vi "Main.vi"() -> ()   [LabVIEW 2017]
uses:
  MassData-Parameter/Utility/Def-MassData Status Indicator(Vertical).ctl
  <userlib>/_NEVSTOP/Communicable State Machine(CSM)/_Polymophic/Add State(s) to Queue By BOOL(Element).vi
  92441261-0e8a-4c49-872b-6a8cc16470f8.vi
  cdca145a-d193-4db9-b465-521fbe583cf5.vi
  <vilib>/Analysis/2dsp.llb/Real FFT.vi
  <userlib>/_NEVSTOP/Communicable State Machine(CSM)/AdvanceAPI/CSM - Revert Arguments-Safe String.vi
  <userlib>/_NEVSTOP/Communicable State Machine(CSM)/AdvanceAPI/CSM - Make String Arguments Safe.vi
  <userlib>/_NEVSTOP/Communicable State Machine(CSM)/AdvanceAPI/CSM - Break Down Multiple States String.vi
  <userlib>/_NEVSTOP/Communicable State Machine(CSM)/AdvanceAPI/CSM - Compact Multiple States.vi
  <userlib>/_NEVSTOP/Communicable State Machine(CSM)/AdvanceAPI/CSM - Keywords.vi
  <userlib>/_NEVSTOP/Communicable State Machine(CSM)/_Shared/Trim Single-line Text.vi
  MassData-Parameter/_support/FGV-MassData.vi
  MassData-Parameter/CSM MassData Parameter Support.lvlib
  <vilib>/Analysis/NI_AALPro.lvlib
  <userlib>/_NEVSTOP/Communicable State Machine(CSM)/Communicable State Machine.lvlib
panel:
  out "MassData Status":T1={"w"={287840.0, 276144.0}, "r"={287840.0, 276144.0}} {"r" scale=1.0..1000000.0 scale format="%#_6p"; "w" scale=1.0..1000000.0 scale format="%#_6p"}
  out "fft":dbl[](graph)
  in  "Gen?":bool
  in  "DataSize":i32=1000
  out "Waveform Chart":dbl[](graph)
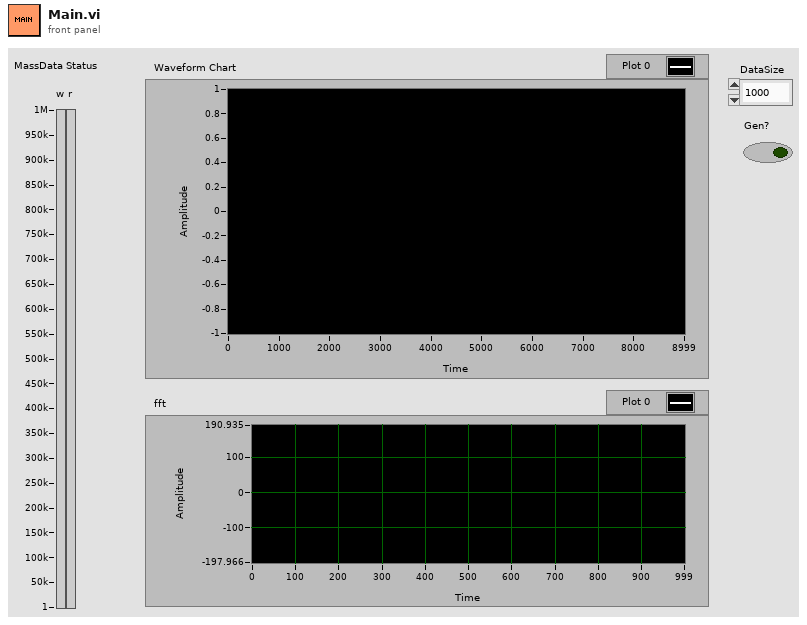
[diagram p1: front panel]
types:
  T1 = typedef "Def-MassData Status Indicator(Vertical).ctl" = cluster{"w":cluster{dbl, dbl}, "r":cluster{dbl, dbl}}
  T2 = enum32{"Invalid", "Standard", "Closed", "Hidden", "Minimized", "Maximized"}
  T3 = enum32{"invalid app kind", "Development System", "Run Time System", "Student Edition", "Embedded LabVIEW", "Evaluation", "Custom"}
  T4 = typedef "Communicable State Machine.lvlib/_CSM_Response Source Message.ctl" = cluster{"‘State":string, "’Arguments":string, "’Error":errorcluster}
  T5 = cluster{"Core":cluster{"Current VI Reference":refnum<vi>, "Close Panel on Exit?":bool}, "Your Boolean data":bool, "Your string data":string}
  T6 = cluster{"Current VI Reference":refnum<vi>, "Close Panel on Exit?":bool}
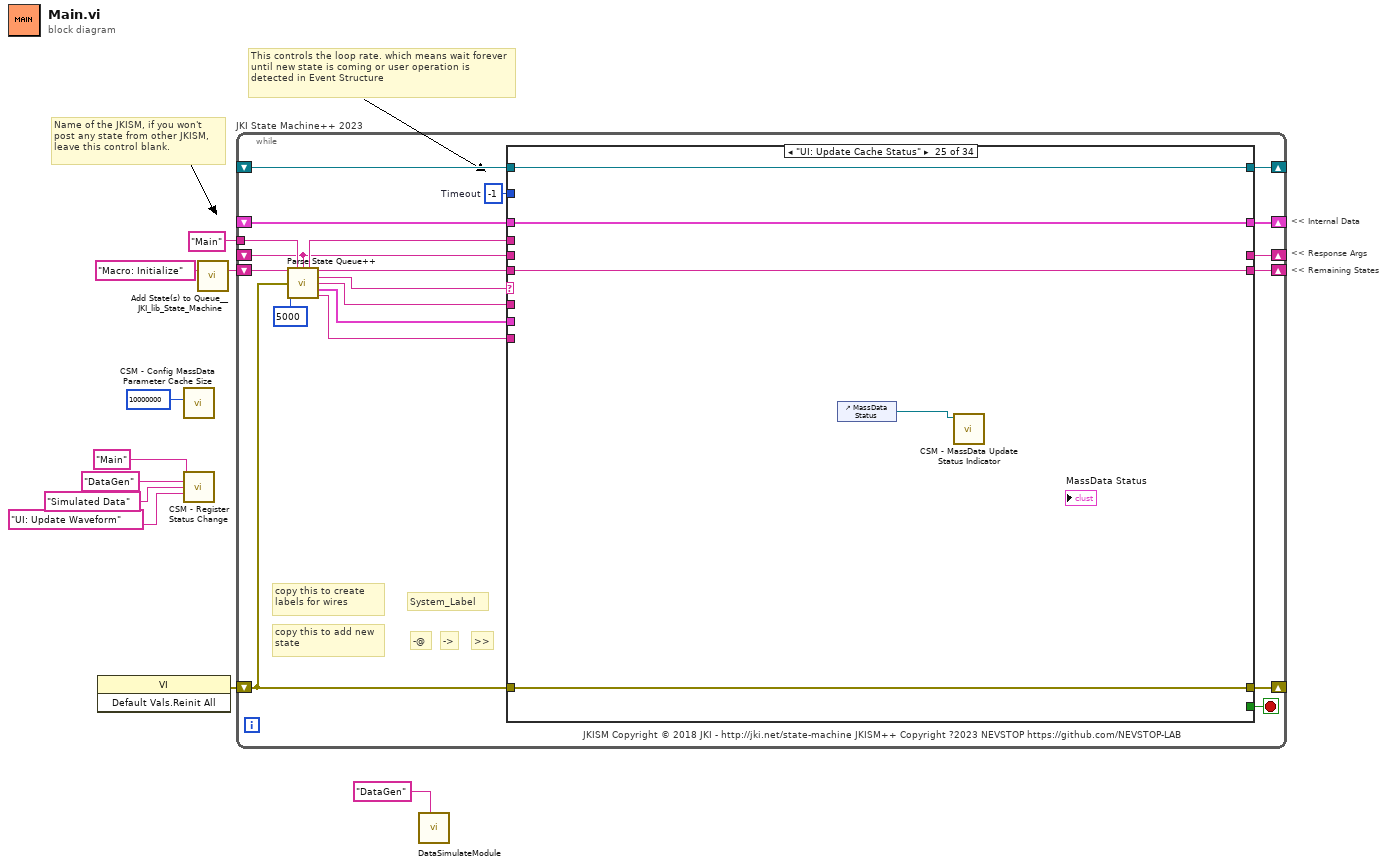
[diagram p0: block diagram]
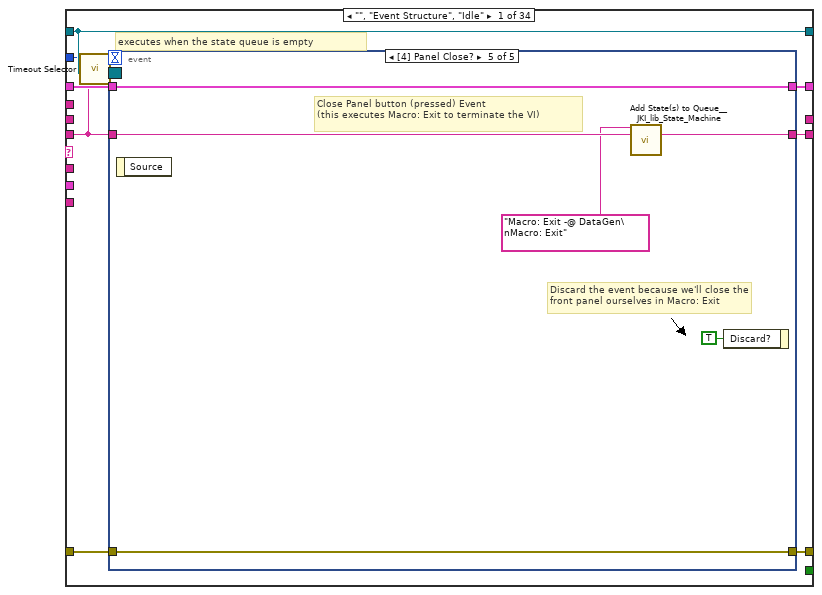
[diagram p2: hidden frame]
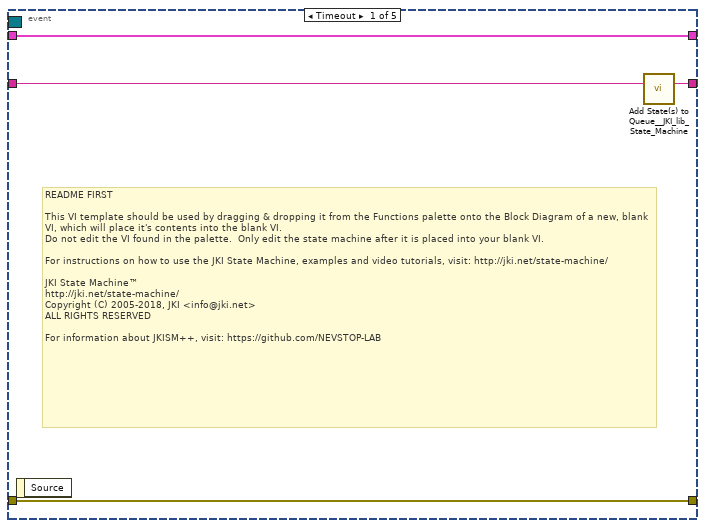
[diagram p3: hidden frame]
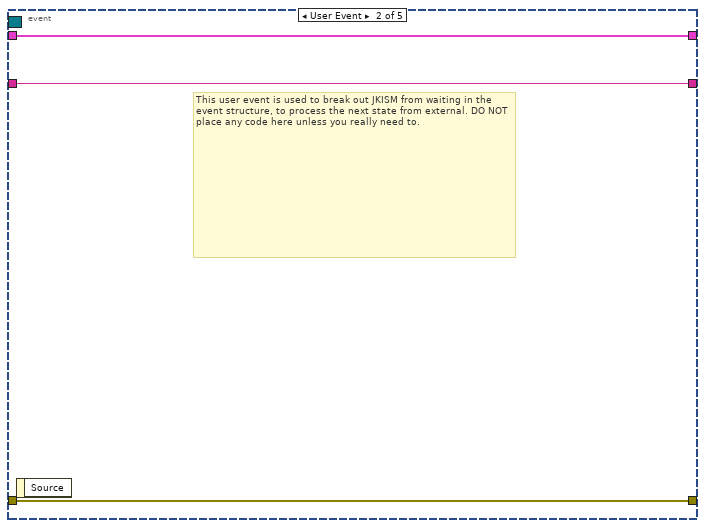
[diagram p4: hidden frame]
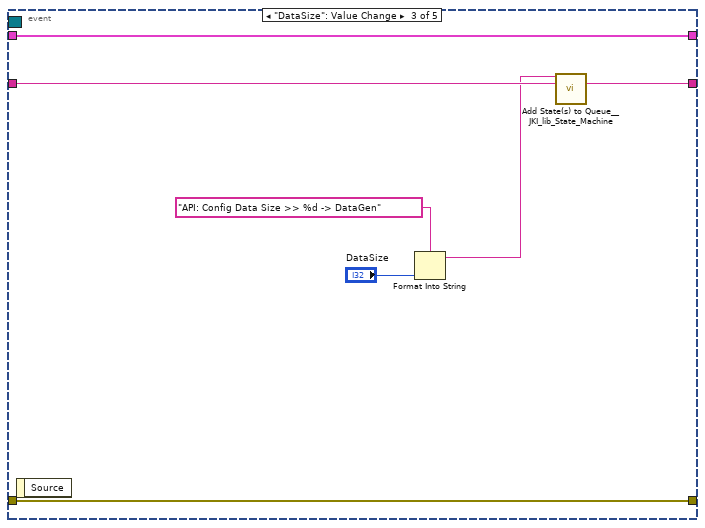
[diagram p5: hidden frame]
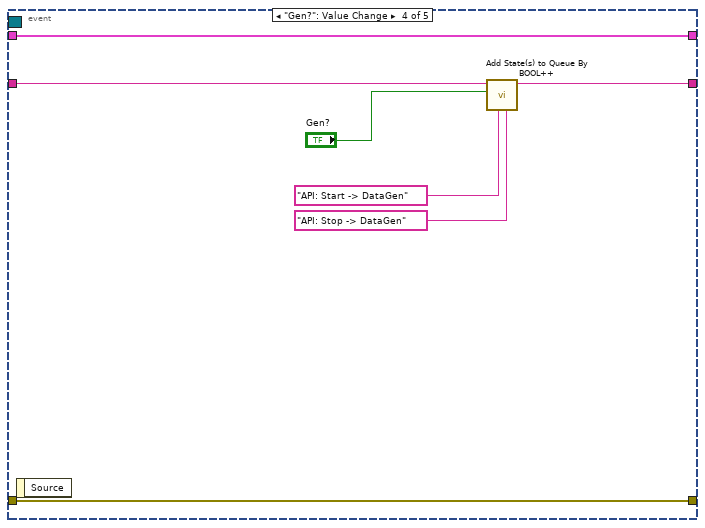
[diagram p6: hidden frame]
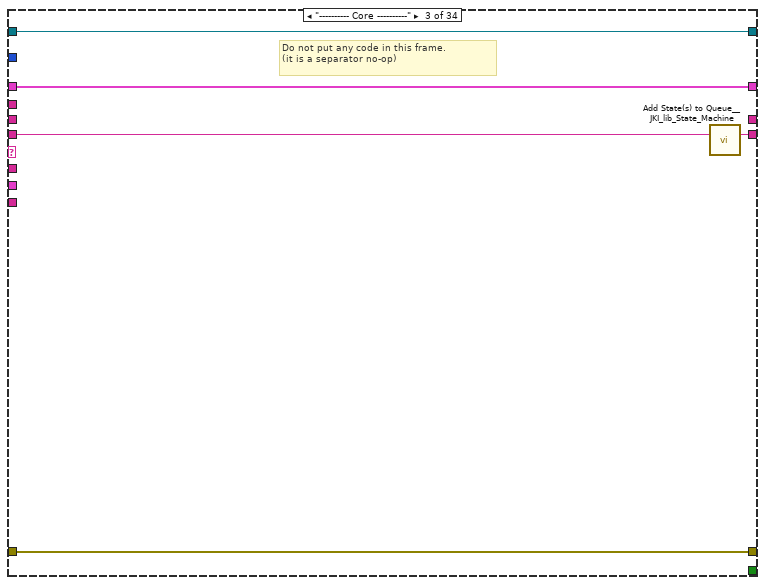
[diagram p8: hidden frame]
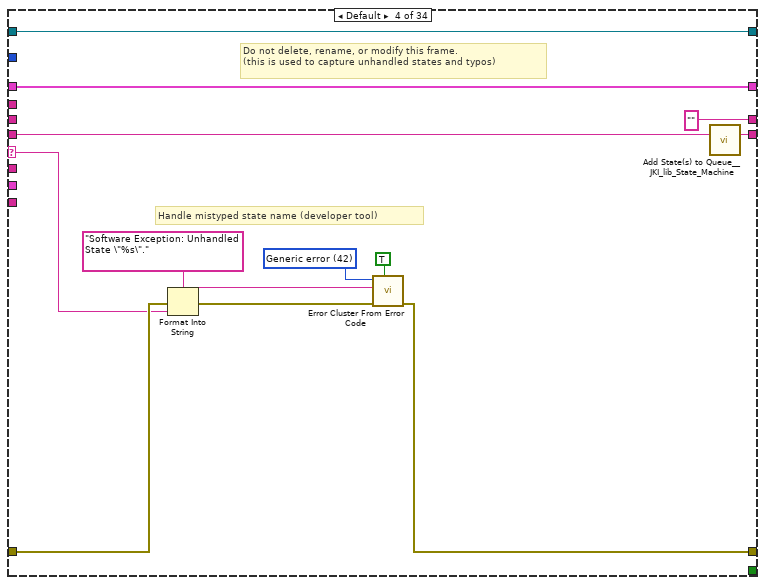
[diagram p9: hidden frame]
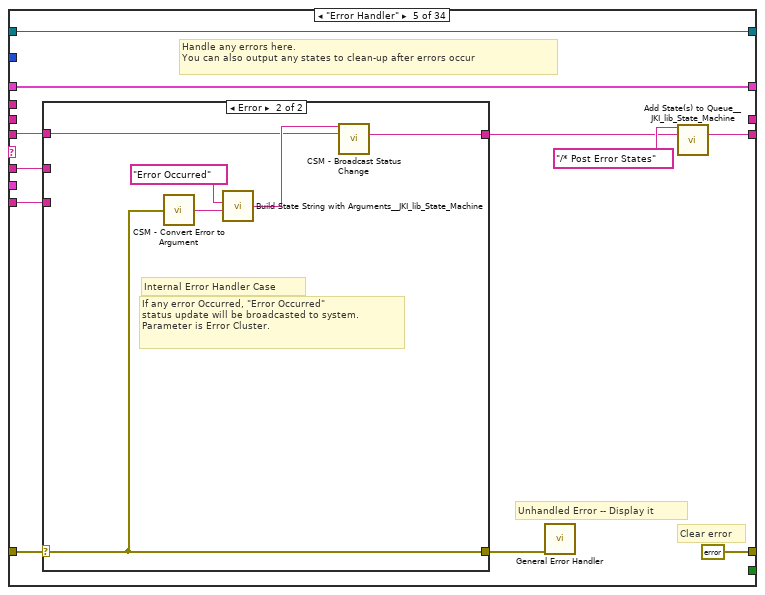
[diagram p10: hidden frame]
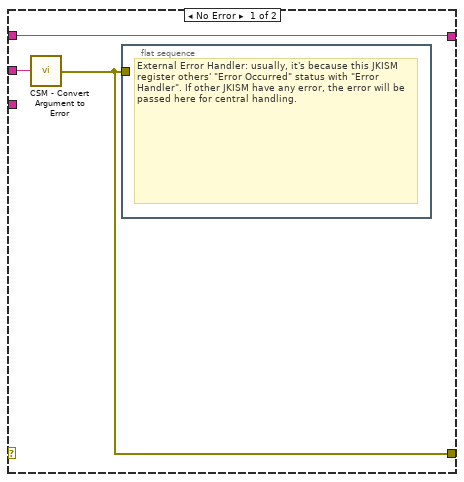
[diagram p11: hidden frame]
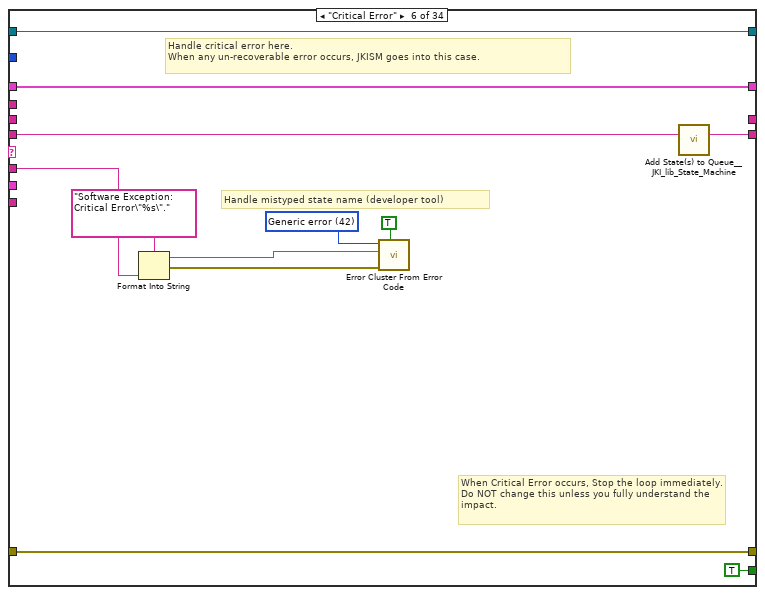
[diagram p12: hidden frame]
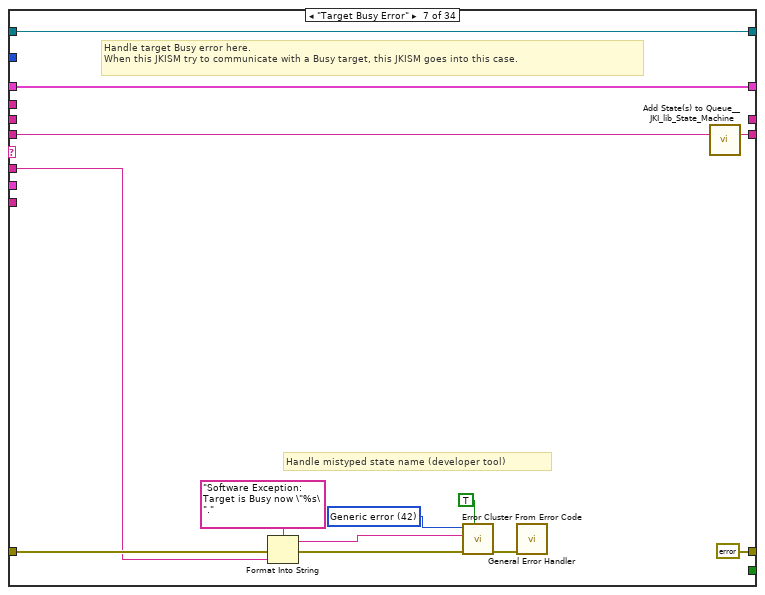
[diagram p13: hidden frame]
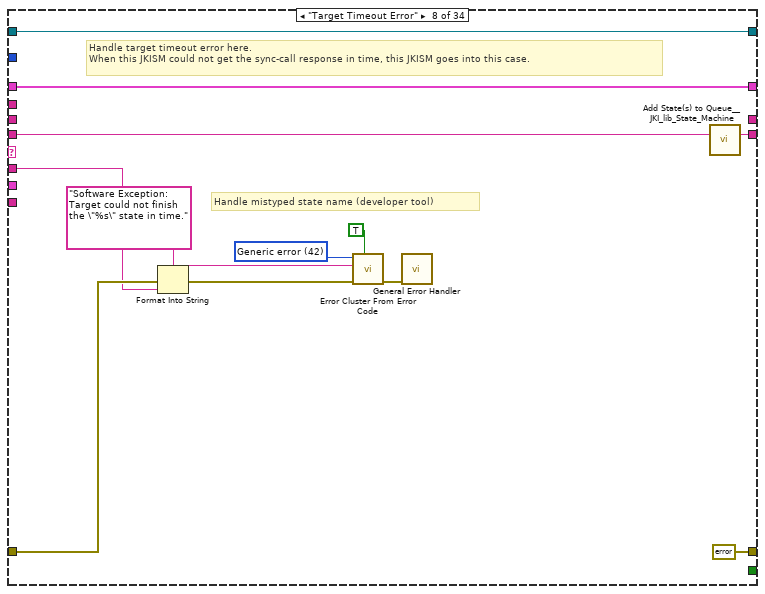
[diagram p14: hidden frame]
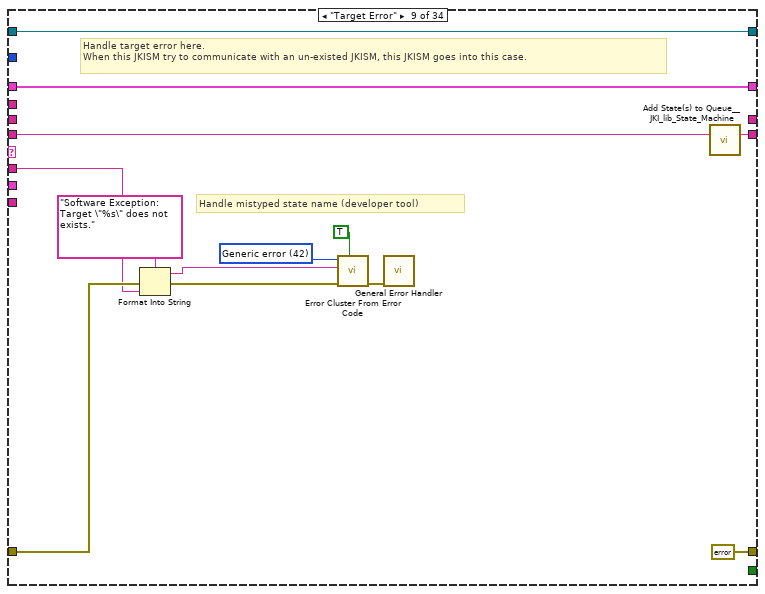
[diagram p15: hidden frame]
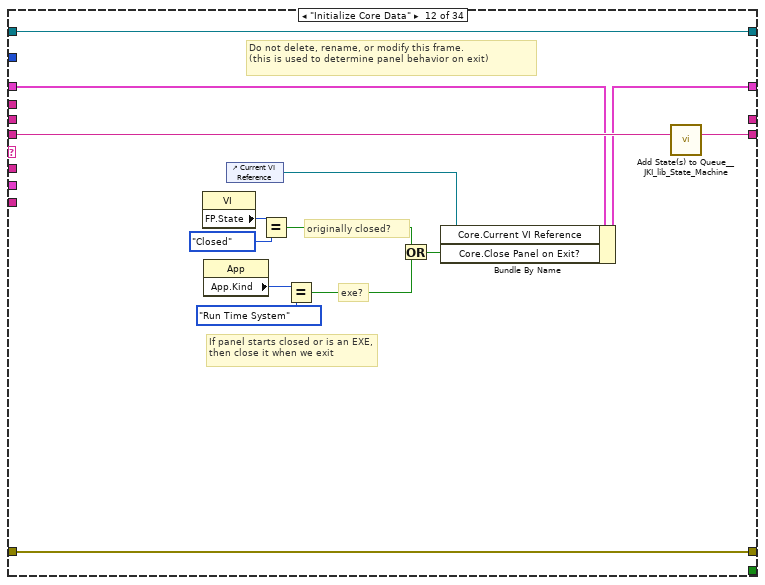
[diagram p18: hidden frame]
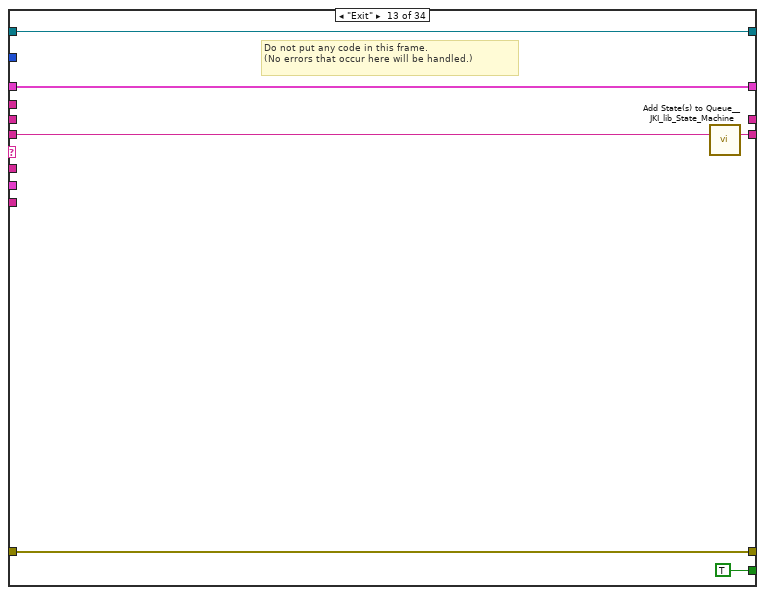
[diagram p19: hidden frame]
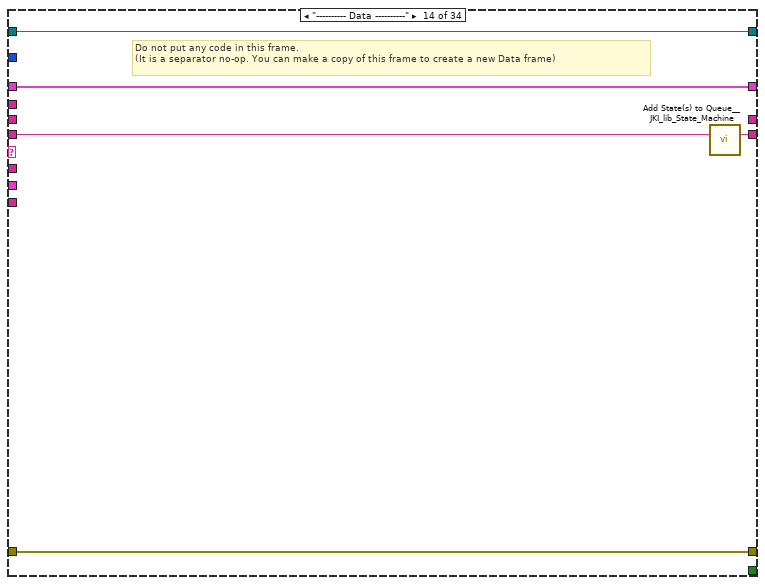
[diagram p20: hidden frame]
diagram:
  # "<< Internal Data"
  # "<< Response Args"
  # "<< Remaining States"
  # "Name of the JKISM, if you won't post any state from other JKISM,  leave this control blank."
  # "This controls the loop rate. which means wait forever until new state is coming or user operation is detected in Event Structure"
  n1 = invoke class="VI" method="Default Vals.Reinit All"() -> (error out=w2:errorcluster)  [unwired: 3 in, 2 out]
  n2 = call "CSM - Config MassData Parameter Cache Size.vi"("size(1M)"=10000000) -> ()  [unwired: 10 in, 1 out]
  n3 = call <userlib>:"CSM - Register Status Change.vi"("CSM Name"="Main" ("JKISM Name"), "Source CSM Name (* as Default)"="DataGen" ("JKISM Name"), "Status"="Simulated Data" ("JKISM Name"), "Response Message (if \"\", same as Source Message)"="UI: Update Waveform" ("JKISM Name")) -> ()  [unwired: 10 in, 2 out]
  n4 = call <vilib>:"Add State(s) to Queue__JKI_lib_State_Machine.vi"("State(s) in (\"\")"="Macro: Initialize") -> ("States Out"=w8:string)  [unwired: 14 in]
  n5 = while "JKI State Machine++ 2023" {
    shift-right: [w25] -> _
    shift-left: _ -> [w24]
    shift-right: [w28] -> _
    shift-left: w2 -> [w22]
    shift-right: [w27] -> _
    shift-left: w8 -> [w29]
    tunnel: "Main" ("Name(\"\" to use uuid)") -> [w17]
    shift-right: [w20] -> _
    shift-left: _ -> [w12]
    shift-right: [w19] -> _
    shift-left: _ -> [w18]
    stop <- w26 stop-if-true
    w23 = -1  # Timeout
    # "JKISM Copyright © 2018 JKI - http://jki.net/state-machine JKISM++ Copyright ?2023 NEVSTOP https://github.com/NEVSTOP-LAB"
    # "copy this to add new state"
    # ">>"
    # "->"
    # "-@"
    # "copy this to create labels for wires"
    # "System_Label"
    n6 = call <userlib>:"Parse State Queue++.vi"("State Queue"=w29, "Name(\"\" to use uuid)"=w17, "Response Arguments"=w12, "Previous Error"=w22, "Response Timeout(-2 use global Settings)"=5000 ("Response Timeout(1000ms)")) -> ("Name Used"=w13:string, "Remaining States"=w30:string, "Current State"=w16:string, "Arguments"=w11:string, ">> Response Source Message >>"=w15:T4, ">> Source CSM >>"=w14:string)  [unwired: 5 in]
    n7 = case shown="\"UI: Update Cache Status\"" w16 {
      selector: w16 -> [_ _ _ w78 _ _ _ _ _ _ _ _ _ _ _ _ _ _ _ _ _ _ _ _ _ _ _ _ _ _ _ _ _ _]
      tunnel: w30 -> [w31 w69 w75 w82 w92 w118 w123 w141 w154 w162 w166 w181 w187 w192 w200 w207 w212 w218 w222 w228 w233 w240 w256 w328 w336 w345 w351 w357 w368 w371 w376 w382 w388 w394]
      tunnel: w11 -> [_ _ _ _ w90 w111 w125 w137 w150 _ _ _ _ _ _ _ _ _ _ _ _ w235 w250 w323 _ w339 _ _ _ _ _ _ _ _]
      tunnel: w24 -> [w38 w68 w72 w80 w98 w119 w127 w139 w152 w161 w165 w174 w185 w189 _ w202 w209 w217 w221 w225 w231 w238 w252 w331 w335 w344 w348 w354 w365 w370 w375 w379 w385 w391]
      tunnel: [w37 w70 w73 w84 errorcluster {"status"=FALSE, "code"=0, "source"=""} ("error out") w120 errorcluster {"status"=FALSE, "code"=0, "source"=""} ("error out") errorcluster {"status"=FALSE, "code"=0, "source"=""} ("error out") errorcluster {"status"=FALSE, "code"=0, "source"=""} ("error out") w163 w167 w178 w184 w190 w197 w203 w210 w213 w220 w226 w230 w236 w253 w332 w337 w346 w349 w355 w366 w372 w377 w380 w386 w392] -> w28
      tunnel: w22 -> [w36 w70 w73 w83 w96 w120 w129 w142 w155 w163 w167 w178 w184 w190 w197 w204 w210 _ w223 w226 w230 w237 w254 w332 w337 w346 w349 w355 w366 w372 w377 w380 w386 w392]
      tunnel: [w39 w69 w74 w81 w94 w117 w128 w140 w153 w162 w166 w180 w186 w191 w199 w206 w211 w218 w222 w227 w232 w239 w255 w329 w336 w345 w350 w356 w367 w371 w376 w381 w387 w393] -> w27
      tunnel: [_ _ _ _ _ TRUE _ _ _ _ _ _ TRUE _ _ _ _ _ _ _ _ _ _ _ _ _ _ _ _ _ _ _ _ _] -> w26
      tunnel: [w35 w68 w72 w80 w98 w119 w127 w139 w152 w161 w165 w179 w185 w189 w198 w202 w209 w217 w221 w225 w231 w238 w252 w331 w335 w344 w348 w354 w365 w370 w375 w379 w385 w391] -> w25
      tunnel: w23 -> [w33 _ _ _ _ _ _ _ _ _ _ _ _ _ _ _ _ _ _ _ _ _ _ _ _ _ _ _ _ _ _ _ _ _]
      tunnel: w14 -> [_ _ _ _ w89 _ _ _ _ _ _ _ _ _ _ _ _ _ _ _ _ _ _ _ _ _ _ _ _ _ _ _ _ _]
      tunnel: w15 -> [_ _ _ _ _ _ _ _ _ _ _ _ _ _ _ _ _ _ _ _ _ _ _ _ _ _ _ _ _ _ _ _ _ _]
      tunnel: [_ _ _ "" _ _ _ _ _ _ _ _ _ _ _ _ _ _ _ _ _ _ _ _ _ _ _ _ _ _ "API1 Response" _ "DoA Finished" "DoB Finished"] -> w20
      tunnel: [w34 w67 w71 w76 w97 w109 w124 w136 w149 w160 w164 w168 w182 w188 w193 w201 w208 w216 w219 w224 w229 w234 w249 w330 w334 w343 w347 w352 w358 w369 w374 w378 w384 w390] -> w19
      tunnel: w18 -> [w34 w67 w71 w76 w97 w109 w124 w136 w149 w160 w164 w168 w182 w188 w193 w201 w208 _ w219 w224 w229 w234 w249 w330 w334 w343 w347 w352 w358 w369 w374 w378 w384 w390]
      tunnel: w13 -> [_ _ _ _ _ _ _ _ _ _ _ _ _ _ _ _ _ w215 _ _ _ _ _ _ _ _ _ _ _ _ _ _ _ _]
      tunnel: w12 -> [_ _ _ _ _ _ _ _ _ _ _ _ _ _ _ _ _ _ _ _ _ _ _ _ _ _ _ _ _ _ _ _ _ _]
      frame "", "Event Structure", "Idle" {
        # "executes when the state queue is empty"
        n8 = call <userlib>:"Timeout Selector.vi"("Remaining States"=w31, "Timeout Expected"=w33) -> ("Timeout"=w32:i32)  [unwired: 5 in]
        n9 = event shown="[4] Panel Close?" {
          selector: w34 -> [_ _ _ _ _]
          dyn-events: _ -> [_ _ _ _ _]
          timeout: w32 -> [_ _ _ _ _]
          tunnel: w31 -> [w43 w45 w50 w57 w66]
          tunnel: [w42 w45 w51 w58 w65] -> w39
          tunnel: w38 -> [w40 w46 w52 w59 w63]
          tunnel: [w41 w44 w53 w60 w64] -> w37
          tunnel: w36 -> [w41 w44 w53 w60 w64]
          tunnel: [w40 w46 w52 w59 w63] -> w35
          event Timeout {
            # "README FIRST\n \nThis VI template should be used by dragging & dropping it from the Functions palette onto the Block Diagram of a new, blank VI, which will place it's contents into the blank VI. \nDo not edit the VI found in the palette.  Only edit the state machine after it is placed into your blank VI.\n \nFor instructions on how to use the JKI State Machine, examples and video tutorials, visit: http://jki.net/state-machine/\n\nJKI State Machine™\nhttp://jki.net/state-machine/\nCopyright (C) 2005-2018, JKI <info@jki.net>\nALL RIGHTS RESERVED\n\nFor information about JKISM++, visit: https://github.com/NEVSTOP-LAB"
            n10 = event-data() -> ()  [unwired: 1 in, 1 out]
            n11 = call <vilib>:"Add State(s) to Queue__JKI_lib_State_Machine.vi"("State(s) in (\"\")"=w43) -> ("States Out"=w42:string)  [unwired: 14 in]
          }
          event User Event {
            # "This user event is used to break out JKISM from waiting in the event structure, to process the next state from external. DO NOT place any code here unless you really need to."
            n12 = event-data() -> ()  [unwired: 1 in, 1 out]
          }
          event "DataSize": Value Change {
            n13 = event-data() -> ()  [unwired: 1 in, 1 out]
            n14 = Format Into String(format string="API: Config Data Size >> %d -> DataGen" ("State(s) in Front (\"\")"), "DataSize") -> (resulting string=w48:string)  [unwired: 2 in, 1 out]
            n15 = call <vilib>:"Add State(s) to Queue__JKI_lib_State_Machine.vi"("State(s) in Front (\"\")"=w48, "State(s) in (\"\")"=w50) -> ("States Out"=w51:string)  [unwired: 13 in]
          }
          event "Gen?": Value Change {
            n16 = event-data() -> ()  [unwired: 1 in, 1 out]
            n17 = call-poly <userlib>:"Add State(s) to Queue By BOOL++.vi"("FALSE(\"\")"="API: Stop -> DataGen" ("TRUE(\"\")"), "TRUE(\"\")"="API: Start -> DataGen" ("TRUE(\"\")"), "Condition"="Gen?", "State Queue(\"\")"=w57) -> ("Remaining States"=w58:string)  [unwired: 7 in]
          }
          event Panel Close? {
            # "Discard the event because we'll close the front panel ourselves in Macro: Exit"
            # "Close Panel button (pressed) Event\n(this executes Macro: Exit to terminate the VI)"
            n18 = event-data() -> ()  [unwired: 1 in, 1 out]
            n19 = call <vilib>:"Add State(s) to Queue__JKI_lib_State_Machine.vi"("State(s) in Front (\"\")"="Macro: Exit -@ DataGen\nMacro: Exit", "State(s) in (\"\")"=w66) -> ("States Out"=w65:string)  [unwired: 13 in]
            n20 = event-data("Discard?"=TRUE) -> ()  [unwired: 1 in, 1 out]
          }
        }
      }
      frame "JKISM++ Documentation" {
        # "JKISM++ Documentation"
        # "State Syntax:\nStateCategory: State >> Argument -@ JKISMName\nStateCategory: State >> Argument -> JKISMName\n\nLine Terminator: Line feed"
        # "Commenting:\nTo add a comment use \"//\" or \"#\" and all text to the right will be ignored\nCommenting Example:\nUI: Initialize // This initializes the UI\n// Another comment line"
        # "Example:\nUI: Help >> About -@Main\nUI: Help >> About ->Main\n\nWhere \"UI\" is the state category\nWhere \"Help\" is the state\nWhere \"About\" is the argument\nWhere \"Main\" is the Name of JKISM,which actually run the \"UI: Help >> About\"\n\n    \"-@\" stands for sync state. Current JKISM will wait until the state is finished. \n            - if \"Main\" named JKISM does not exist, \"Target Error\" will occur.\n            - if \"Main\" named JKISM is in another sync remote state, \"Target Busy Error\" will occur.\n            - if \"Main\" named JKISM could not finish the state in time, \"Target Timeout Error\" will occur.\n            - if everything is right. \"Response\" will occur with Argument back from \"Main\" named JKISM. \n\n    \"->\" stands for async state. Current JKISM will post the state and continue to next state in next iteration.\n            - if \"Main\" named JKISM does not exist, \"Target Error\" will occur.\n            - if everything is right. \"Async Message Posted\" will occur.\n            - After State is finished. Caller will receive a \"Async Response\" state from callee.\n\nWhen duplicated name is used for multiple JKISM module or some framework problem happens, \"Critical Error\" will occur."
      }
      frame "---------- Core ----------" {
        # "Do not put any code in this frame.\n(it is a separator no-op)"
        n21 = call <vilib>:"Add State(s) to Queue__JKI_lib_State_Machine.vi"("State(s) in (\"\")"=w75) -> ("States Out"=w74:string)  [unwired: 14 in]
      }
      frame Default {
        w87 = 42 items=["No error", "Argument error", "Memory is full", "Out of zone", "End of file", "File already open", "Generic file I/O error", "File not found", "File permission error", "Disk is full", "Duplicate path", "Too many files open", "System feature not enabled", "Resource file not found", "Cannot add resource", "Resource not found", "Image not found", "Image memory error", "Pen does not exist", "Config type invalid", "Config token not found", "Config parse error", "Config memory error", "Bad external code format", "Bad external code offset", "External code not present", "Null window", "Destroy window error", "Null menu", "Print aborted", "Bad print record", "Print driver error", "Windows error during printing", "Memory error during printing", "Print dialog error", "Generic print error", "Invalid device refnum", "Device not found", "Device parameter error", "Device unit error", "Cannot open device", "Device call aborted", "Generic error", "Cancelled by user", "Object ID too low", "Object ID too high", "Object not in heap", "Unknown heap", "Unknown object (invalid DefProc)", "Unknown object (DefProc not in table)", "Message out of range", "Invalid (null) method", "Unknown message", "Manager call not supported", "Bad address", "Network operation in progress", "Network operation timed out", "Connection is busy", "Network attribute not supported", "Network error", "Address in use", "System out of memory", "Connection aborted", "Connection refused", "Not connected", "Already connected", "Connection closed", "Initialization error (interapplication manager)", "Bad occurrence", "Wait on unbound occurrence handler", "Occurrence queue overflow", "Datalog type conflict", "Unused", "Unrecognized type (interapplication manager)", "Memory corrupt", "Failed to make temporary DLL", "Old CIN version", "Drag socket not found", "Failed to load drop-object", "Failed to register OLE object", "Failed to release OLE object", "Format specifier type mismatch", "Unknown format specifier", "Too few format specifiers", "Too many format specifiers", "Scan failed", "Newer CIN version", "Error converting to variant", "Runtime menu error", "Password tampered", "Variant attribute not found", "Incompatible variant data type", "Event data is not available", "Event Store is not present", "Occurrence is not found", "Event Queue is not created", "Event info is not available", "Refnum passed is NULL", "Error retrieving Class GUID", "Error retrieving CoClass GUID", "Error retrieving TypeLib GUID.", "Bad built application magic bytes.", "Specific driver is different from the specific driver associated with the Logical Name.", "There is no session opened to the class driver.", "Max Error", "MAX - Error with config objects", "MAX - Error loading configuration", "MAX - Group not supported"]
        # "Do not delete, rename, or modify this frame.\n(this is used to capture unhandled states and typos)"
        # "Handle mistyped state name (developer tool)"
        n22 = Format Into String(format string="Software Exception: Unhandled State \"%s\"." ("message"), error in=w83, w78) -> (resulting string=w86:string, error out=w85:errorcluster)  [unwired: 1 in]
        n23 = call <vilib>:"Error Cluster From Error Code.vi"("show call chain? (False)"=TRUE, "error in (no error)"=w85, "error message (\"\")"=w86, "error code (0)"=w87) -> ("error out"=w84:errorcluster)  [unwired: 5 in]
        n24 = call <vilib>:"Add State(s) to Queue__JKI_lib_State_Machine.vi"("State(s) in (\"\")"=w82) -> ("States Out"=w81:string)  [unwired: 14 in]
      }
      frame "Error Handler" {
        # "Unhandled Error -- Display it"
        # "Handle any errors here.\nYou can also output any states to clean-up after errors occur"
        # "Clear error"
        n25 = case shown="Error" w96 {
          selector: w96 -> [_ w103]
          tunnel: [w101 w105] -> w93
          tunnel: w92 -> [w101 w104]
          tunnel: [w100 w103] -> w91
          tunnel: w90 -> [w102 _]
          tunnel: w89 -> [_ _]
          frame No Error {
            n26 = call <userlib>:"CSM - Convert Argument to Error.vi"("Argument"=w102) -> ("error"=w100:errorcluster)  [unwired: 4 in]
            n27 = flat-sequence {
              tunnel: w100 -> [_]
              frame #0 {
                # "External Error Handler: usually, it's because this JKISM register others' \"Error Occurred\" status with \"Error Handler\". If other JKISM have any error, the error will be passed here for central handling."
              }
            }
          }
          frame Error {
            # "Internal Error Handler Case"
            # "If any error Occurred, \"Error Occurred\" \nstatus update will be broadcasted to system.\nParameter is Error Cluster."
            n28 = call <userlib>:"CSM - Convert Error to Argument.vi"("error"=w103) -> ("Argument"=w107:string)  [unwired: 4 in]
            n29 = call <vilib>:"Build State String with Arguments__JKI_lib_State_Machine.vi"("Arguments (\"\")"=w107, "State"="Error Occurred" ("Status with Arguments")) -> ("State with Arguments"=w106:string)  [unwired: 4 in]
            n30 = call <userlib>:"CSM - Broadcast Status Change.vi"("Status with Arguments"=w106, "State Queue"=w104) -> ("Remaining States"=w105:string)  [unwired: 13 in]
          }
        }
        n31 = call <vilib>:"General Error Handler.vi"("error in (no error)"=w91) -> ()  [unwired: 10 in, 5 out]
        n32 = call <vilib>:"Add State(s) to Queue__JKI_lib_State_Machine.vi"("State(s) in Front (\"\")"="/* Post Error States", "State(s) in (\"\")"=w93) -> ("States Out"=w94:string)  [unwired: 13 in]
      }
      frame "Critical Error" {
        w115 = 42 items=["No error", "Argument error", "Memory is full", "Out of zone", "End of file", "File already open", "Generic file I/O error", "File not found", "File permission error", "Disk is full", "Duplicate path", "Too many files open", "System feature not enabled", "Resource file not found", "Cannot add resource", "Resource not found", "Image not found", "Image memory error", "Pen does not exist", "Config type invalid", "Config token not found", "Config parse error", "Config memory error", "Bad external code format", "Bad external code offset", "External code not present", "Null window", "Destroy window error", "Null menu", "Print aborted", "Bad print record", "Print driver error", "Windows error during printing", "Memory error during printing", "Print dialog error", "Generic print error", "Invalid device refnum", "Device not found", "Device parameter error", "Device unit error", "Cannot open device", "Device call aborted", "Generic error", "Cancelled by user", "Object ID too low", "Object ID too high", "Object not in heap", "Unknown heap", "Unknown object (invalid DefProc)", "Unknown object (DefProc not in table)", "Message out of range", "Invalid (null) method", "Unknown message", "Manager call not supported", "Bad address", "Network operation in progress", "Network operation timed out", "Connection is busy", "Network attribute not supported", "Network error", "Address in use", "System out of memory", "Connection aborted", "Connection refused", "Not connected", "Already connected", "Connection closed", "Initialization error (interapplication manager)", "Bad occurrence", "Wait on unbound occurrence handler", "Occurrence queue overflow", "Datalog type conflict", "Unused", "Unrecognized type (interapplication manager)", "Memory corrupt", "Failed to make temporary DLL", "Old CIN version", "Drag socket not found", "Failed to load drop-object", "Failed to register OLE object", "Failed to release OLE object", "Format specifier type mismatch", "Unknown format specifier", "Too few format specifiers", "Too many format specifiers", "Scan failed", "Newer CIN version", "Error converting to variant", "Runtime menu error", "Password tampered", "Variant attribute not found", "Incompatible variant data type", "Event data is not available", "Event Store is not present", "Occurrence is not found", "Event Queue is not created", "Event info is not available", "Refnum passed is NULL", "Error retrieving Class GUID", "Error retrieving CoClass GUID", "Error retrieving TypeLib GUID.", "Bad built application magic bytes.", "Specific driver is different from the specific driver associated with the Logical Name.", "There is no session opened to the class driver.", "Max Error", "MAX - Error with config objects", "MAX - Error loading configuration", "MAX - Group not supported"]
        # "Handle critical error here.\nWhen any un-recoverable error occurs, JKISM goes into this case."
        # "When Critical Error occurs, Stop the loop immediately. Do NOT change this unless you fully understand the impact."
        # "Handle mistyped state name (developer tool)"
        n33 = Format Into String(format string="Software Exception: Critical Error\"%s\"." ("message"), w111) -> (resulting string=w114:string, error out=w113:errorcluster)  [unwired: 2 in]
        n34 = call <vilib>:"Error Cluster From Error Code.vi"("show call chain? (False)"=TRUE, "error in (no error)"=w113, "error message (\"\")"=w114, "error code (0)"=w115) -> ()  [unwired: 5 in, 1 out]
        n35 = call <vilib>:"Add State(s) to Queue__JKI_lib_State_Machine.vi"("State(s) in (\"\")"=w118) -> ("States Out"=w117:string)  [unwired: 14 in]
      }
      frame "Target Busy Error" {
        w132 = 42 items=["No error", "Argument error", "Memory is full", "Out of zone", "End of file", "File already open", "Generic file I/O error", "File not found", "File permission error", "Disk is full", "Duplicate path", "Too many files open", "System feature not enabled", "Resource file not found", "Cannot add resource", "Resource not found", "Image not found", "Image memory error", "Pen does not exist", "Config type invalid", "Config token not found", "Config parse error", "Config memory error", "Bad external code format", "Bad external code offset", "External code not present", "Null window", "Destroy window error", "Null menu", "Print aborted", "Bad print record", "Print driver error", "Windows error during printing", "Memory error during printing", "Print dialog error", "Generic print error", "Invalid device refnum", "Device not found", "Device parameter error", "Device unit error", "Cannot open device", "Device call aborted", "Generic error", "Cancelled by user", "Object ID too low", "Object ID too high", "Object not in heap", "Unknown heap", "Unknown object (invalid DefProc)", "Unknown object (DefProc not in table)", "Message out of range", "Invalid (null) method", "Unknown message", "Manager call not supported", "Bad address", "Network operation in progress", "Network operation timed out", "Connection is busy", "Network attribute not supported", "Network error", "Address in use", "System out of memory", "Connection aborted", "Connection refused", "Not connected", "Already connected", "Connection closed", "Initialization error (interapplication manager)", "Bad occurrence", "Wait on unbound occurrence handler", "Occurrence queue overflow", "Datalog type conflict", "Unused", "Unrecognized type (interapplication manager)", "Memory corrupt", "Failed to make temporary DLL", "Old CIN version", "Drag socket not found", "Failed to load drop-object", "Failed to register OLE object", "Failed to release OLE object", "Format specifier type mismatch", "Unknown format specifier", "Too few format specifiers", "Too many format specifiers", "Scan failed", "Newer CIN version", "Error converting to variant", "Runtime menu error", "Password tampered", "Variant attribute not found", "Incompatible variant data type", "Event data is not available", "Event Store is not present", "Occurrence is not found", "Event Queue is not created", "Event info is not available", "Refnum passed is NULL", "Error retrieving Class GUID", "Error retrieving CoClass GUID", "Error retrieving TypeLib GUID.", "Bad built application magic bytes.", "Specific driver is different from the specific driver associated with the Logical Name.", "There is no session opened to the class driver.", "Max Error", "MAX - Error with config objects", "MAX - Error loading configuration", "MAX - Group not supported"]
        # "Handle target Busy error here.\nWhen this JKISM try to communicate with a Busy target, this JKISM goes into this case."
        # "Handle mistyped state name (developer tool)"
        n36 = Format Into String(format string="Software Exception: Target is Busy now \"%s\"." ("message"), error in=w129, w125) -> (resulting string=w131:string, error out=w130:errorcluster)  [unwired: 1 in]
        n37 = call <vilib>:"Error Cluster From Error Code.vi"("show call chain? (False)"=TRUE, "error in (no error)"=w130, "error message (\"\")"=w131, "error code (0)"=w132) -> ("error out"=w122:errorcluster)  [unwired: 5 in]
        n38 = call <vilib>:"General Error Handler.vi"("error in (no error)"=w122) -> ()  [unwired: 10 in, 5 out]
        n39 = call <vilib>:"Add State(s) to Queue__JKI_lib_State_Machine.vi"("State(s) in (\"\")"=w123) -> ("States Out"=w128:string)  [unwired: 14 in]
      }
      frame "Target Timeout Error" {
        w145 = 42 items=["No error", "Argument error", "Memory is full", "Out of zone", "End of file", "File already open", "Generic file I/O error", "File not found", "File permission error", "Disk is full", "Duplicate path", "Too many files open", "System feature not enabled", "Resource file not found", "Cannot add resource", "Resource not found", "Image not found", "Image memory error", "Pen does not exist", "Config type invalid", "Config token not found", "Config parse error", "Config memory error", "Bad external code format", "Bad external code offset", "External code not present", "Null window", "Destroy window error", "Null menu", "Print aborted", "Bad print record", "Print driver error", "Windows error during printing", "Memory error during printing", "Print dialog error", "Generic print error", "Invalid device refnum", "Device not found", "Device parameter error", "Device unit error", "Cannot open device", "Device call aborted", "Generic error", "Cancelled by user", "Object ID too low", "Object ID too high", "Object not in heap", "Unknown heap", "Unknown object (invalid DefProc)", "Unknown object (DefProc not in table)", "Message out of range", "Invalid (null) method", "Unknown message", "Manager call not supported", "Bad address", "Network operation in progress", "Network operation timed out", "Connection is busy", "Network attribute not supported", "Network error", "Address in use", "System out of memory", "Connection aborted", "Connection refused", "Not connected", "Already connected", "Connection closed", "Initialization error (interapplication manager)", "Bad occurrence", "Wait on unbound occurrence handler", "Occurrence queue overflow", "Datalog type conflict", "Unused", "Unrecognized type (interapplication manager)", "Memory corrupt", "Failed to make temporary DLL", "Old CIN version", "Drag socket not found", "Failed to load drop-object", "Failed to register OLE object", "Failed to release OLE object", "Format specifier type mismatch", "Unknown format specifier", "Too few format specifiers", "Too many format specifiers", "Scan failed", "Newer CIN version", "Error converting to variant", "Runtime menu error", "Password tampered", "Variant attribute not found", "Incompatible variant data type", "Event data is not available", "Event Store is not present", "Occurrence is not found", "Event Queue is not created", "Event info is not available", "Refnum passed is NULL", "Error retrieving Class GUID", "Error retrieving CoClass GUID", "Error retrieving TypeLib GUID.", "Bad built application magic bytes.", "Specific driver is different from the specific driver associated with the Logical Name.", "There is no session opened to the class driver.", "Max Error", "MAX - Error with config objects", "MAX - Error loading configuration", "MAX - Group not supported"]
        # "Handle target timeout error here.\nWhen this JKISM could not get the sync-call response in time, this JKISM goes into this case."
        # "Handle mistyped state name (developer tool)"
        n40 = Format Into String(format string="Software Exception: Target could not finish the \"%s\" state in time." ("message"), error in=w142, w137) -> (resulting string=w144:string, error out=w143:errorcluster)  [unwired: 1 in]
        n41 = call <vilib>:"Error Cluster From Error Code.vi"("show call chain? (False)"=TRUE, "error in (no error)"=w143, "error message (\"\")"=w144, "error code (0)"=w145) -> ("error out"=w134:errorcluster)  [unwired: 5 in]
        n42 = call <vilib>:"General Error Handler.vi"("error in (no error)"=w134) -> ()  [unwired: 10 in, 5 out]
        n43 = call <vilib>:"Add State(s) to Queue__JKI_lib_State_Machine.vi"("State(s) in (\"\")"=w141) -> ("States Out"=w140:string)  [unwired: 14 in]
      }
      frame "Target Error" {
        w158 = 42 items=["No error", "Argument error", "Memory is full", "Out of zone", "End of file", "File already open", "Generic file I/O error", "File not found", "File permission error", "Disk is full", "Duplicate path", "Too many files open", "System feature not enabled", "Resource file not found", "Cannot add resource", "Resource not found", "Image not found", "Image memory error", "Pen does not exist", "Config type invalid", "Config token not found", "Config parse error", "Config memory error", "Bad external code format", "Bad external code offset", "External code not present", "Null window", "Destroy window error", "Null menu", "Print aborted", "Bad print record", "Print driver error", "Windows error during printing", "Memory error during printing", "Print dialog error", "Generic print error", "Invalid device refnum", "Device not found", "Device parameter error", "Device unit error", "Cannot open device", "Device call aborted", "Generic error", "Cancelled by user", "Object ID too low", "Object ID too high", "Object not in heap", "Unknown heap", "Unknown object (invalid DefProc)", "Unknown object (DefProc not in table)", "Message out of range", "Invalid (null) method", "Unknown message", "Manager call not supported", "Bad address", "Network operation in progress", "Network operation timed out", "Connection is busy", "Network attribute not supported", "Network error", "Address in use", "System out of memory", "Connection aborted", "Connection refused", "Not connected", "Already connected", "Connection closed", "Initialization error (interapplication manager)", "Bad occurrence", "Wait on unbound occurrence handler", "Occurrence queue overflow", "Datalog type conflict", "Unused", "Unrecognized type (interapplication manager)", "Memory corrupt", "Failed to make temporary DLL", "Old CIN version", "Drag socket not found", "Failed to load drop-object", "Failed to register OLE object", "Failed to release OLE object", "Format specifier type mismatch", "Unknown format specifier", "Too few format specifiers", "Too many format specifiers", "Scan failed", "Newer CIN version", "Error converting to variant", "Runtime menu error", "Password tampered", "Variant attribute not found", "Incompatible variant data type", "Event data is not available", "Event Store is not present", "Occurrence is not found", "Event Queue is not created", "Event info is not available", "Refnum passed is NULL", "Error retrieving Class GUID", "Error retrieving CoClass GUID", "Error retrieving TypeLib GUID.", "Bad built application magic bytes.", "Specific driver is different from the specific driver associated with the Logical Name.", "There is no session opened to the class driver.", "Max Error", "MAX - Error with config objects", "MAX - Error loading configuration", "MAX - Group not supported"]
        # "Handle target error here.\nWhen this JKISM try to communicate with an un-existed JKISM, this JKISM goes into this case."
        # "Handle mistyped state name (developer tool)"
        n44 = Format Into String(format string="Software Exception: Target \"%s\" does not exists." ("message"), error in=w155, w150) -> (resulting string=w157:string, error out=w156:errorcluster)  [unwired: 1 in]
        n45 = call <vilib>:"Error Cluster From Error Code.vi"("show call chain? (False)"=TRUE, "error in (no error)"=w156, "error message (\"\")"=w157, "error code (0)"=w158) -> ("error out"=w148:errorcluster)  [unwired: 5 in]
        n46 = call <vilib>:"General Error Handler.vi"("error in (no error)"=w148) -> ()  [unwired: 10 in, 5 out]
        n47 = call <vilib>:"Add State(s) to Queue__JKI_lib_State_Machine.vi"("State(s) in (\"\")"=w154) -> ("States Out"=w153:string)  [unwired: 14 in]
      }
      frame "Async Response", "Response" {
        # "Handle Async-call Response (\"Async Response\" for ->)"
        # "Handle Sync-call Response (\"Response\" for -@)"
        # "After Message is executed, JKISM+ goes to this state for receive the response. \n    For Async Message(->), \"Async Response\" is used. This JKISM will goes to \"Async Message Posted\" immediately and receive the \"Async Response\" after the callee finishes the message.\n    For Sync Message(@),  This JKISM will wait until the message is done and immediately goes to \"Response\""
      }
      frame "Async Message Posted" {
        # "Handle post action for async message (->)."
        # "After Async Message is posted (->), JKISM+ goes to this state for post-action. You can use Argument - State to tell which Async Message is called."
      }
      frame "Initialize Core Data" {
        # "Do not delete, rename, or modify this frame.\n(this is used to determine panel behavior on exit)"
        # "originally closed?"
        # "exe?"
        # "If panel starts closed or is an EXE, then close it when we exit"
        n48 = property class="VI"() -> ("FP.State"=w171:T2)  [unwired: 2 in, 2 out]
        n49 = property class="App"() -> ("App.Kind"=w177:T3)  [unwired: 2 in, 2 out]
        n50 = control-ref of="Current VI Reference"() -> (w172:refnum<vi>)
        n51 = Equal?(x=w171, y=T2."Closed" ("Front Panel Window:State")) -> (x = y?=w169:bool)
        n52 = Equal?(x=w177, y=T3."Run Time System" ("Application:Kind")) -> (x = y?=w175:bool)
        n53 = Or(x=w169, y=w175) -> (x .or. y?=w173:bool)
        n54 = Bundle By Name(cluster=w174, "Core.Current VI Reference"=w172, "Core.Close Panel on Exit?"=w173) -> (w179:T5)
        n55 = call <vilib>:"Add State(s) to Queue__JKI_lib_State_Machine.vi"("State(s) in (\"\")"=w181) -> ("States Out"=w180:string)  [unwired: 14 in]
      }
      frame "Exit" {
        # "Do not put any code in this frame.\n(No errors that occur here will be handled.)"
        n56 = call <vilib>:"Add State(s) to Queue__JKI_lib_State_Machine.vi"("State(s) in (\"\")"=w187) -> ("States Out"=w186:string)  [unwired: 14 in]
      }
      frame "---------- Data ----------" {
        # "Do not put any code in this frame.\n(It is a separator no-op. You can make a copy of this frame to create a new Data frame)"
        n57 = call <vilib>:"Add State(s) to Queue__JKI_lib_State_Machine.vi"("State(s) in (\"\")"=w192) -> ("States Out"=w191:string)  [unwired: 14 in]
      }
      frame "Data: Initialize" {
        w194 = T6 {"Current VI Reference"=refnum, "Close Panel on Exit?"=FALSE}  # Core
        w196 = TRUE  # Your Boolean data
        w195 = ""  # Your string data
        # "do not delete - used by framework"
        # "Expand Bundle to add new data elements to shift register data."
        # "Add new data here."
        # "Data names and types of shift register data are defined by this bundle."
        # "Initialize the shift-register data, here.\n(data names are defined by what you wire into the bundle function)"
        n58 = Bundle("Core"=w194, "Your Boolean data"=w196, "Your string data"=w195) -> (w198:T5)  [unwired: 1 in]
        n59 = call <vilib>:"Add State(s) to Queue__JKI_lib_State_Machine.vi"("State(s) in (\"\")"=w200) -> ("States Out"=w199:string)  [unwired: 14 in]
      }
      frame "Data: Cleanup" {
        # "Cleanup any data and references, here.\n(this is called automatically, by the Macro: Exit)"
        n60 = Unbundle By Name(w202) -> ("Core.Current VI Reference"=w205:refnum<vi>)
        n61 = Close Reference(reference=w205, error in (no error)=w204) -> (error out=w203:errorcluster)
        n62 = call <vilib>:"Add State(s) to Queue__JKI_lib_State_Machine.vi"("State(s) in (\"\")"=w207) -> ("States Out"=w206:string)  [unwired: 14 in]
      }
      frame "---------- Events ----------" {
        # "Do not put any code in this frame.\n(It is a separator no-op. You can make a copy of this frame to create a new UI frame)"
        n63 = call <vilib>:"Add State(s) to Queue__JKI_lib_State_Machine.vi"("State(s) in (\"\")"=w212) -> ("States Out"=w211:string)  [unwired: 14 in]
      }
      frame "Events: Register" {
        # "Register message event to break Waiting in Event structure."
        n64 = call <userlib>:"CSM - Get New State Notifier Event.vi"("Name(\"\" to use uuid) in"=w215) -> ("Error out"=w213:errorcluster, "New State Notifier Event"=w214:refnum<user-event>)  [unwired: 9 in]
        n65 = register-events(w214) -> (reference out=w216:refnum<event-registration>)  [unwired: 2 in, 1 out]
      }
      frame "Events: Unregister" {
        n66 = Unregister For Events(event registration refnum=w219, error in=w223) -> (error out=w220:errorcluster)
      }
      frame "---------- UI ----------" {
        # "Do not put any code in this frame.\n(It is a separator no-op. You can make a copy of this frame to create a new UI frame)"
        n67 = call <vilib>:"Add State(s) to Queue__JKI_lib_State_Machine.vi"("State(s) in (\"\")"=w228) -> ("States Out"=w227:string)  [unwired: 14 in]
      }
      frame "UI: Initialize" {
        # "Initialize the User Interface, here.\n(this is called automatically, by the Macro: Init)"
        n68 = call <vilib>:"Add State(s) to Queue__JKI_lib_State_Machine.vi"("State(s) in (\"\")"=w233) -> ("States Out"=w232:string)  [unwired: 14 in]
      }
      frame "UI: Cursor Set" {
        # "Argument"
        # "Set and Unset Cursor Busy.\n(Usage: \"UI: Cursor Set >> Busy|Idle\")"
        n69 = disable-structure shown="Default" {
          disable-tunnel: w237 -> [w243 w248]
          disable-tunnel: [w242 w248] -> w236
          disable-tunnel: w235 -> [w241 _]
          frame condition #0 (active) {
            n70 = case shown="\"Busy\"" w241 {
              tunnel: w243 -> [w245 w247]
              tunnel: [w244 w246] -> w242
              frame "Idle", Default {
                n71 = call <vilib>:"Unset Busy.vi"("error in (no error)"=w245) -> ("error out"=w244:errorcluster)  [unwired: 10 in]
              }
              frame "Busy" {
                n72 = call <vilib>:"Set Busy.vi"("error in (no error)"=w247) -> ("error out"=w246:errorcluster)  [unwired: 9 in, 1 out]
              }
            }
          }
          frame condition #1 {
          }
        }
        n73 = call <vilib>:"Add State(s) to Queue__JKI_lib_State_Machine.vi"("State(s) in (\"\")"=w240) -> ("States Out"=w239:string)  [unwired: 14 in]
      }
      frame "UI: Front Panel State" {
        # "Argument"
        # "Set Front Panel Open or Closed\n(Usage: \"UI: Front Panel State >> Open|Close\")"
        n74 = Unbundle By Name(w252) -> ("Core.Current VI Reference"=w251:refnum<vi>)
        n75 = case shown="\"Minimize\", \"Minimized\"" w250 {
          tunnel: w254 -> [w262 w277 w288 w301 w314]
          tunnel: [w264 w278 w290 w303 w316] -> w253
          tunnel: w251 -> [w263 w275 w289 w302 w315]
          frame "Open", "Standard", Default {
            w257 = T2."Standard" ("State")
            n76 = property class="VI"(reference=w263, error in=w262) -> (reference out=w260:refnum<vi>, error out=w261:errorcluster, "FP.State"=w259:T2)
            n77 = Not Equal?(x=w259, y=w257) -> (x != y?=w258:bool)
            n78 = case shown="True" w258 {
              tunnel: [w268 w270] -> w264
              tunnel: w261 -> [w267 w270]
              tunnel: w260 -> [w266 _]
              tunnel: w257 -> [w265 _]
              frame True {
                n79 = invoke class="VI" method="FP.Open"(reference=w266, error in=w267, "Activate"=TRUE, "State"=w265) -> (error out=w268:errorcluster)  [unwired: 1 in, 4 out]
              }
              frame False {
              }
            }
          }
          frame "Close", "Closed" {
            n80 = property class="VI"(reference=w275, error in=w277) -> (reference out=w274:refnum<vi>, error out=w276:errorcluster, "FP.State"=w272:T2)
            n81 = Not Equal?(x=w272, y=T2."Closed" ("Front Panel Window:State")) -> (x != y?=w271:bool)
            n82 = case shown="True" w271 {
              tunnel: [w279 w282] -> w278
              tunnel: w276 -> [w279 w281]
              tunnel: w274 -> [_ w280]
              frame False {
              }
              frame True {
                n83 = invoke class="VI" method="FP.Close"(reference=w280, error in=w281) -> (error out=w282:errorcluster)  [unwired: 1 in, 2 out]
              }
            }
          }
          frame "Hidden", "Hide" {
            w283 = T2."Hidden" ("State")
            n84 = property class="VI"(reference=w289, error in=w288) -> (reference out=w286:refnum<vi>, error out=w287:errorcluster, "FP.State"=w285:T2)
            n85 = Not Equal?(x=w285, y=w283) -> (x != y?=w284:bool)
            n86 = case shown="True" w284 {
              tunnel: [w294 w295] -> w290
              tunnel: w287 -> [w293 w295]
              tunnel: w286 -> [w292 _]
              tunnel: w283 -> [w291 _]
              frame True {
                n87 = invoke class="VI" method="FP.Open"(reference=w292, error in=w293, "State"=w291) -> (error out=w294:errorcluster)  [unwired: 2 in, 4 out]
              }
              frame False {
              }
            }
          }
          frame "Minimize", "Minimized" {
            w296 = T2."Minimized" ("State")
            n88 = property class="VI"(reference=w302, error in=w301) -> (reference out=w299:refnum<vi>, error out=w300:errorcluster, "FP.State"=w298:T2)
            n89 = Not Equal?(x=w298, y=w296) -> (x != y?=w297:bool)
            n90 = case shown="True" w297 {
              tunnel: [w307 w308] -> w303
              tunnel: w300 -> [w306 w308]
              tunnel: w299 -> [w305 _]
              tunnel: w296 -> [w304 _]
              frame True {
                n91 = invoke class="VI" method="FP.Open"(reference=w305, error in=w306, "State"=w304) -> (error out=w307:errorcluster)  [unwired: 2 in, 4 out]
              }
              frame False {
              }
            }
          }
          frame "Maximize", "Maximized" {
            w309 = T2."Maximized" ("State")
            n92 = property class="VI"(reference=w315, error in=w314) -> (reference out=w312:refnum<vi>, error out=w313:errorcluster, "FP.State"=w311:T2)
            n93 = Not Equal?(x=w311, y=w309) -> (x != y?=w310:bool)
            n94 = case shown="True" w310 {
              tunnel: [w320 w321] -> w316
              tunnel: w313 -> [w319 w321]
              tunnel: w312 -> [w318 _]
              tunnel: w309 -> [w317 _]
              frame True {
                n95 = invoke class="VI" method="FP.Open"(reference=w318, error in=w319, "State"=w317) -> (error out=w320:errorcluster)  [unwired: 2 in, 4 out]
              }
              frame False {
              }
            }
          }
        }
        n96 = call <vilib>:"Add State(s) to Queue__JKI_lib_State_Machine.vi"("State(s) in (\"\")"=w256) -> ("States Out"=w255:string)  [unwired: 14 in]
      }
      frame "UI: Update Waveform" {
        n97 = call "CSM - Convert Argument to MassData.vim"("Type"=dbl[] [], "MassData Argument"=w323) -> ("Data"=→"Waveform Chart":dbl[])  [unwired: 6 in, 1 out]
        n98 = call <vilib>:"Build State String with Arguments__JKI_lib_State_Machine.vi"("Arguments (\"\")"=w323, "State"="UI: FFT" ("State(s) in Front (\"\")")) -> ("State with Arguments"=w326:string)  [unwired: 4 in]
        n99 = call <vilib>:"Add State(s) to Queue__JKI_lib_State_Machine.vi"("State(s) in Front (\"\")"=w326, "State(s) in (\"\")"=w328, "State(s) at Back (\"\")"="UI: Update Cache Status" ("State(s) at Back (\"\")")) -> ("States Out"=w329:string)  [unwired: 12 in]
      }
      frame "UI: Update Cache Status" {
        n100 = control-ref of="MassData Status"() -> (w333:refnum<vi>)
        n101 = call "CSM - MassData Update Status Indicator.vi"("MassData Status Indicator"=w333) -> ()  [unwired: 10 in, 1 out]
      }
      frame "UI: FFT" {
        n102 = call "CSM - Convert Argument to MassData.vim"("Type"=dbl[] [], "MassData Argument"=w339) -> ("Data"=w338:dbl[])  [unwired: 6 in, 1 out]
        n103 = local read "DataSize"() -> (w342:i32)
        n104 = call-poly <vilib>:"FFT.vi"("FFT size"=w342, "X"=w338) -> ("FFT {X}"=→"fft":cdb[])  [unwired: 8 in, 1 out]
      }
      frame "---------- Macro ----------" {
        # "Do not put any code in this frame.\n(It is a separator no-op. You can make a copy of this frame to create a new Macro frame)"
        n105 = call <vilib>:"Add State(s) to Queue__JKI_lib_State_Machine.vi"("State(s) in (\"\")"=w351) -> ("States Out"=w350:string)  [unwired: 14 in]
      }
      frame "Macro: Initialize" {
        w353 = "Data: Initialize\nInitialize Core Data\nEvents: Register\nUI: Initialize\nUI: Front Panel State >> Open"  # Data: Initialize Initialize Core Data Events: Register UI: Initialize UI: Front Panel State >> Open
        # "Initialization Macro\n(This is called once, when the VI starts)"
        n106 = call <vilib>:"Add State(s) to Queue__JKI_lib_State_Machine.vi"("State(s) in Front (\"\")"=w353, "State(s) in (\"\")"=w357) -> ("States Out"=w356:string)  [unwired: 13 in]
      }
      frame "Macro: Exit" {
        # "Exit Macro\n(This is called once, when the VI exits)"
        n107 = Unbundle By Name(w365) -> ("Core.Close Panel on Exit?"=w364:bool)
        n108 = Select(t="UI: Front Panel State >> Close", s=w364, f="") -> (s? t:f=w361:string)
        n109 = call <vilib>:"Add State(s) to Queue__JKI_lib_State_Machine.vi"("State(s) in (\"\")"=w361, "State(s) at Back (\"\")"="Data: Cleanup\nEvents: Unregister\nExit") -> ("States Out"=w359:string)  [unwired: 13 in]
        n110 = call <vilib>:"Add State(s) to Queue__JKI_lib_State_Machine.vi"("State(s) in Front (\"\")"=w359, "State(s) in (\"\")"=w368) -> ("States Out"=w367:string)  [unwired: 13 in]
      }
      frame "---------- API ----------" {
        # "Do not put any code in this frame.\n(It is a separator no-op. This category is recommended to use for external API)"
      }
      frame "API: API1" {
        # "If you need to tell who triggered this state , use this string. If it's this case itself, this string is \"\"."
        # "Deal with the parameter if any"
        # "Connect this to return the response of your API"
        # "Copy/Rename this case for your own API"
      }
      frame "---------- DoSth ----------" {
        # "Template Separator\n(You can make a copy of, or modify, this frame)"
        n111 = call <vilib>:"Add State(s) to Queue__JKI_lib_State_Machine.vi"("State(s) in (\"\")"=w382) -> ("States Out"=w381:string)  [unwired: 14 in]
      }
      frame "DoSth: DoA" {
        # "Your code here.\n(You can make a copy of, or modify, this frame)"
        n112 = call <vilib>:"Add State(s) to Queue__JKI_lib_State_Machine.vi"("State(s) in (\"\")"=w388) -> ("States Out"=w387:string)  [unwired: 14 in]
      }
      frame "DoSth: DoB" {
        # "Your code here.\n(You can make a copy of, or modify, this frame)"
        n113 = call <vilib>:"Add State(s) to Queue__JKI_lib_State_Machine.vi"("State(s) in (\"\")"=w394) -> ("States Out"=w393:string)  [unwired: 14 in]
      }
    }
  }
  n114 = call "DataSimulateModule.vi"("Name(\"\" to use uuid)"="DataGen" ("Name(\"\" to use uuid)")) -> ()  [unwired: 11 in]
